vi "TCP.IP Server for Ripple Detection - for data.vi"() -> ()   [LabVIEW 2021]
doc: "Demonstrates how to set up a basic TCP connection, send data to the specified port once a connection has been established, and terminate the connection once the data has been sent. This VI is designed to stop if the TCP connection is terminated. The data sent in this example is an array of random numbers."
panel:
  out "Waveform Graph 10":dbl[](graph)
  in  "loop 1":i32
  in  "Client Closed":string="The client VI closed the connection."
  in  "Stop":bool
  # "Overview: Demonstrates the use of the TCP functions to initialize a TCP server that can send data to a client VI.\nInstructions:\n1. Run the VI.\n2. Open Simple TCP - Client.vi and follow the instructions on its front panel. Note that if you wait longer than 30 seconds to do this after running this VI, it will time out.\n3. Click Stop to stop the VI. Note that if you stop the client VI, this VI will stop automatically."
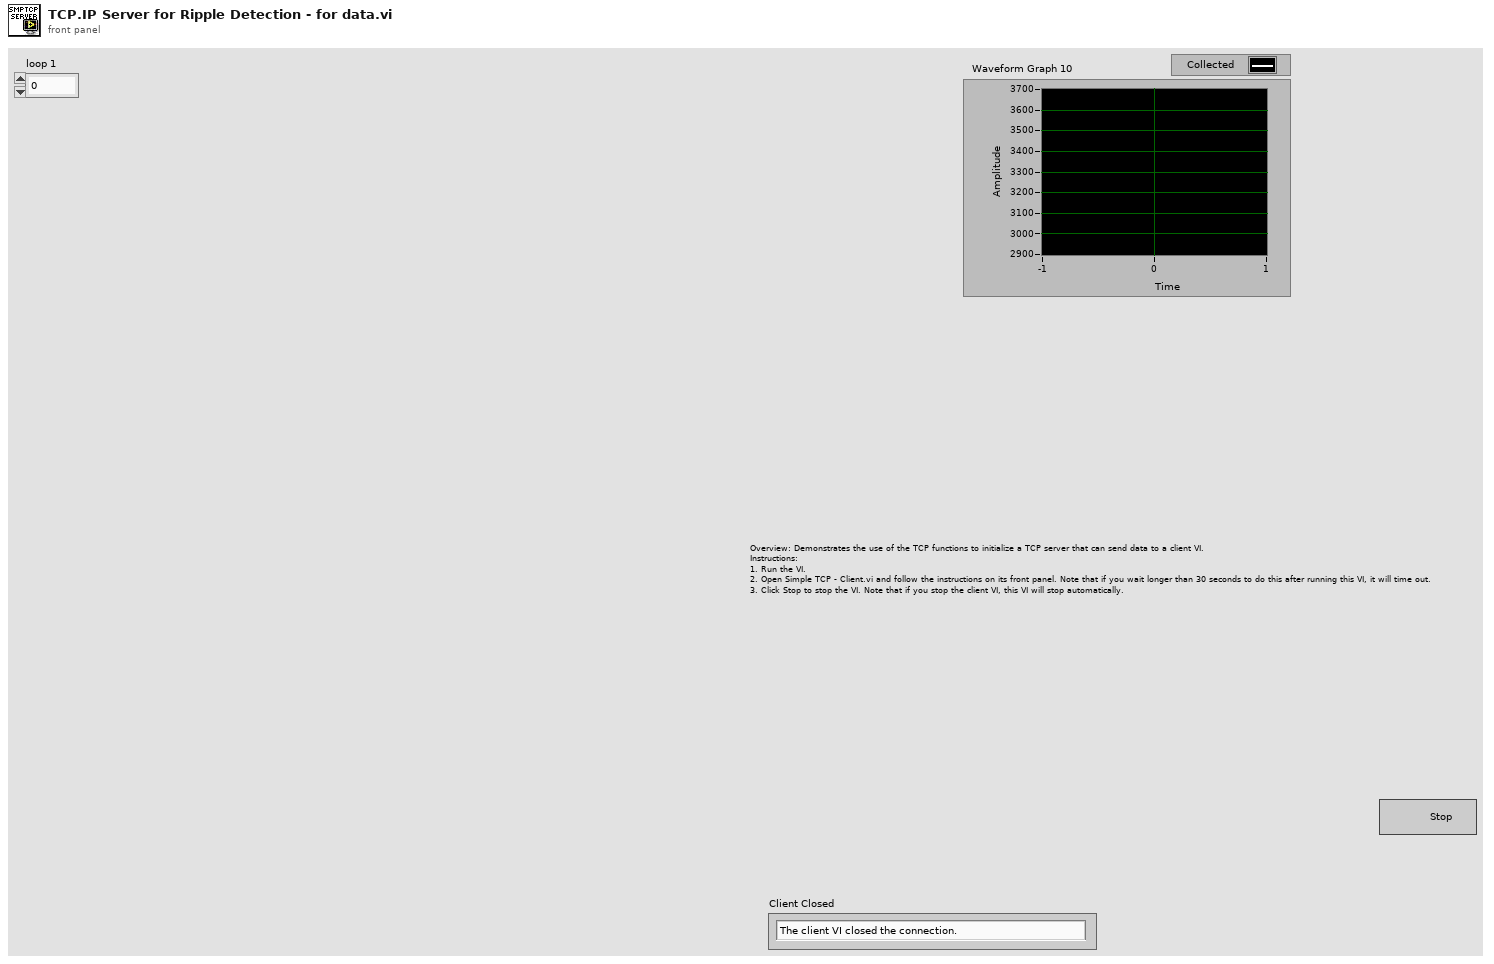
[diagram p1: front panel]
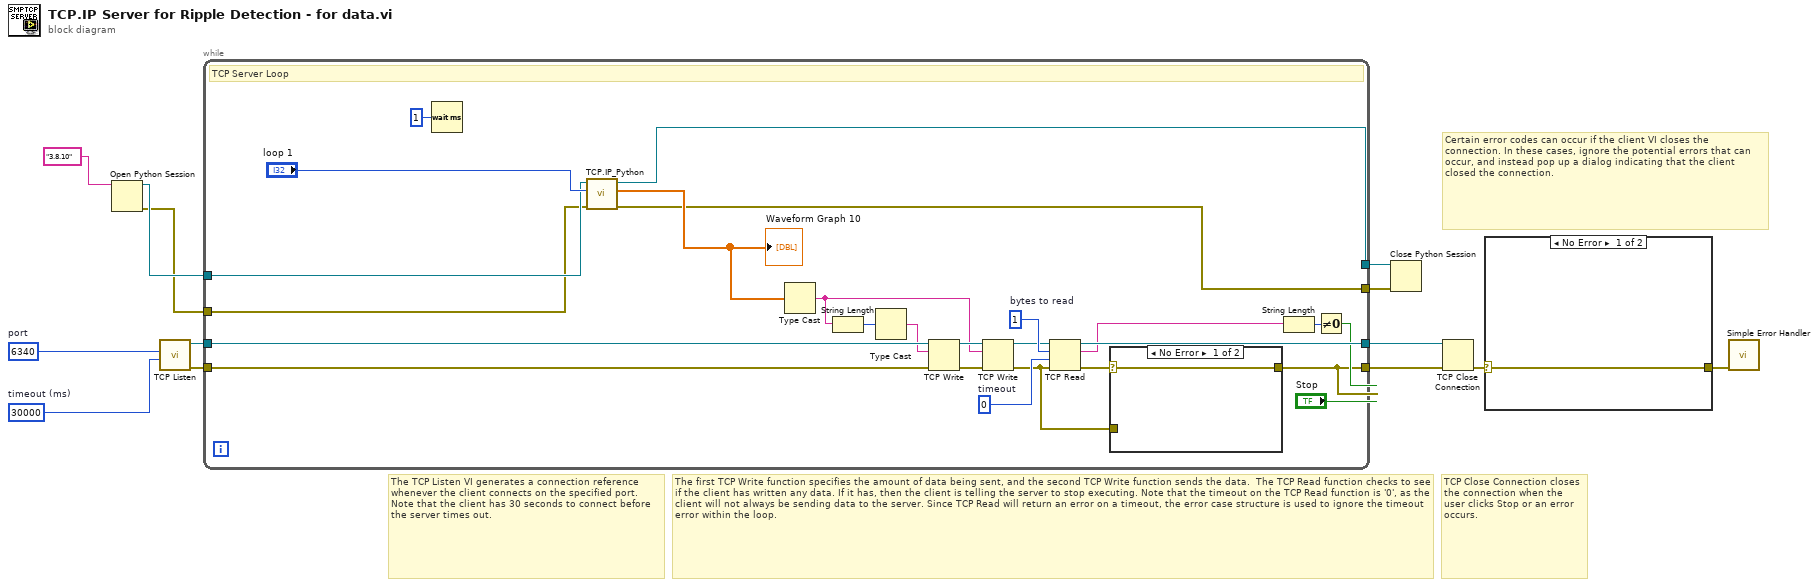
[diagram p0: block diagram]
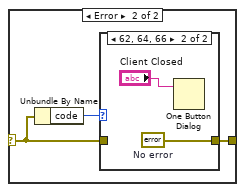
[diagram p2: hidden frame]
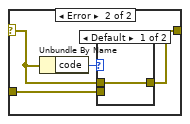
[diagram p4: hidden frame]
diagram:
  w6 = u16 6340  # port
  w7 = 30000  # timeout (ms)
  # "TCP Close Connection closes the connection when the user clicks Stop or an error occurs."
  # "The TCP Listen VI generates a connection reference whenever the client connects on the specified port. Note that the client has 30 seconds to connect before the server times out."
  # "Certain error codes can occur if the client VI closes the connection. In these cases, ignore the potential errors that can occur, and instead pop up a dialog indicating that the client closed the connection."
  # "The first TCP Write function specifies the amount of data being sent, and the second TCP Write function sends the data.  The TCP Read function checks to see if the client has written any data. If it has, then the client is telling the server to stop executing. Note that the timeout on the TCP Read function is '0', as the client will not always be sending data to the server. Since TCP Read will return an error on a timeout, the error case structure is used to ignore the timeout error within the loop."
  n1 = Open Python Session(python version="3.8.10" ("Python version")) -> (session out=w4:refnum<k35>, error out=w3:errorcluster)  [unwired: 2 in]
  n2 = call <vilib>:"TCP Listen.vi"("timeout ms (wait forever: -1)"=w7, "port"=w6) -> ("error out"=w8:errorcluster, "connection ID"=w9:refnum<k5>)  [unwired: 5 in, 3 out]
  n3 = while {
    tunnel: [w22] -> w12
    tunnel: [w28] -> w13
    tunnel: w9 -> [w39]
    tunnel: w8 -> [w32]
    tunnel: w4 -> [w18]
    tunnel: w3 -> [w17]
    tunnel: [w16] -> w2
    tunnel: [w15] -> w1
    stop <- w33 stop-if-true
    w27 = 0  # timeout
    w30 = 1  # bytes to read
    # "TCP Server Loop"
    n4 = Wait (ms)(milliseconds to wait=u32 1) -> ()  [unwired: 1 out]
    n5 = call "TCP.IP_Python.vi"("error in (no error)"=w17, "loop 1"="loop 1", "Refnum in"=w18) -> ("error out"=w15:errorcluster, "Array"=w19:dbl[], "Refnum out"=w16:refnum<k35>)  [unwired: 6 in]
    "Waveform Graph 10" <- w19
    n6 = Type Cast(x=w19) -> (*(type *) &x=w34:string)  [unwired: 1 out]
    n7 = String Length(string=w34) -> (length=w36:i32)
    n8 = Type Cast(x=w36) -> (*(type *) &x=w35:string)  [unwired: 1 out]
    n9 = TCP Write(connection ID=w39, data in=w35, error in (no error)=w32) -> (connection ID out=w38:refnum<k5>, error out=w37:errorcluster)  [unwired: 2 out]
    n10 = TCP Write(connection ID=w38, data in=w34, error in (no error)=w37) -> (connection ID out=w29:refnum<k5>, error out=w21:errorcluster)  [unwired: 2 out]
    n11 = TCP Read(connection ID=w29, bytes to read=w30, error in (no error)=w21, 9:w27) -> (connection ID out=w28:refnum<k5>, data out=w25:string, error out=w23:errorcluster)  [unwired: 1 out]
    n12 = case shown="No Error" w23 {
      selector: w23 -> [w40 w43]
      tunnel: [w40 w41] -> w22
      tunnel: w21 -> [_ w42]
      frame No Error {
      }
      frame Error {
        n13 = Unbundle By Name(w43) -> ("code"=w44:i32)
        n14 = case shown="Default" w44 {
          tunnel: w43 -> [w45 _]
          tunnel: w42 -> [_ w46]
          tunnel: [w45 w46] -> w41
          frame Default {
          }
          frame 56 {
          }
        }
      }
    }
    n15 = String Length(string=w25) -> (length=w26:i32)
    n16 = Not Equal To 0?(x=w26) -> (x != 0?=w24:bool)
    n17 = Compound Arithmetic op=OR(w24, w22, "Stop") -> (w33:bool)
  }
  n18 = Close Python Session(session in=w2, error in=w1) -> ()  [unwired: 1 out]
  n19 = TCP Close Connection(connection ID=w13, error in (no error)=w12) -> (error out=w11:errorcluster)  [unwired: 2 out]
  n20 = case shown="No Error" w11 {
    selector: w11 -> [w47 w49]
    tunnel: [w47 w48] -> w10
    frame No Error {
    }
    frame Error {
      n21 = Unbundle By Name(w49) -> ("code"=w50:i32)
      n22 = case shown="62, 64, 66" w50 {
        tunnel: w49 -> [w51 _]
        tunnel: [w51 w53] -> w48
        frame Default {
        }
        frame 62, 64, 66 {
          w53 = errorcluster {"status"=FALSE, "code"=0, "source"=""}  # No error
          n23 = One Button Dialog(message="Client Closed") -> ()  [unwired: 1 in, 1 out]
        }
      }
    }
  }
  n24 = call <vilib>:"Simple Error Handler.vi"("error in (no error)"=w10) -> ()  [unwired: 1 in, 8 out]
